vi "Begin.vi"(8 "error in (no error)":errorcluster, 9 "Left":T1, 10 "Right":T1, 11 "Pod Drive in":refnum<class "Pod Drive.lvclass">) -> (0 "error out":errorcluster, 3 "Pod Drive out":refnum<class "Pod Drive.lvclass">)   [LabVIEW 2018, in "Drive.lvlib" / "Pod Drive.lvclass"]
doc: "This VI holds the begin code"
uses:
  Pod Drive.lvclass
  Pod.ctl
  <vilib>/Rock Robotics/WPI/SafetyOutput/WPI_SafetyOutputConfigMenu.ctl
  Pod Drive.lvclass/Pod Drive.ctl
  <vilib>/Rock Robotics/WPI/RobotDrive/WPI_RobotDriveOpen2MotorWithExistingMotors.vi
  Drive.lvclass
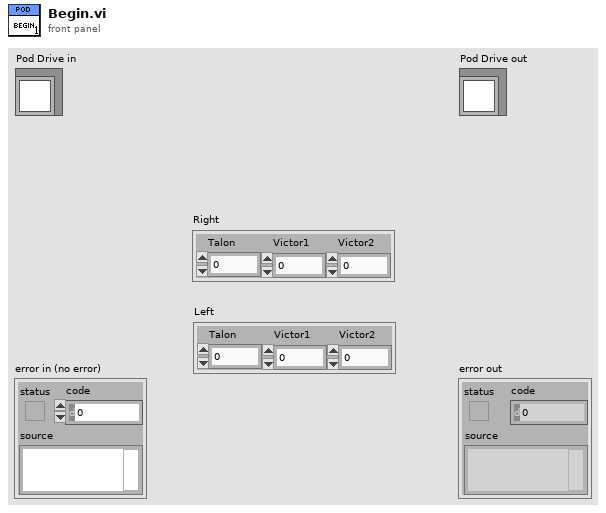
[diagram p1: front panel]
types:
  T1 = typedef "Drive.lvlib/Pod Drive.lvclass/Pod.ctl" = cluster{"Talon":u8, "Victor1":u8, "Victor2":u8}
  T2 = typedef "WPI_SafetyOutputConfigMenu.ctl" = enum16{"Enable", "Disable"}
  T3 = typedef "Drive.lvlib/Drive.lvclass/Drive Sensor Data.ctl" = cluster{"Drive Right Invert":bool, "Drive Right Sensor Phase":bool, "Drive Left Invert":bool, "Drive Left Sensor Phase":bool}
  T4 = typedef "WPI_MotorControlDeviceRef.ctl" = cluster{"DeviceStatus":errorcluster, "Type":T5, "PWM":cluster{"PWM Channel":T6, "DeadBand":T7}, "CAN":cluster{"Device Number":u8, "SetOutput VI Ref":variant, "GetOutput VI Ref":variant, "Enable VI Ref":variant, "Disable VI Ref":variant, "Data":variant}, "Invert":bool, "DIO PWM":cluster{"PWM \"Enable\" Channel":T6, "DIOChannel":T8, "PWM Rate":dbl}}
  T5 = typedef "WPI_MotorControlType.ctl" = enum16{"PWM", "CAN", "DIO PWM"}
  T6 = typedef "FPGA_DIOPWMChannel.ctl" = enum8{"PWM 0", "PWM 1", "PWM 2", "PWM 3", "PWM 4", "PWM 5", "PWM 6", "PWM 7", "PWM 8", "PWM 9", "PWM MXP 0", "PWM MXP 1", "PWM MXP 2", "PWM MXP 3", "PWM MXP 4", "PWM MXP 5", "PWM MXP 6", "PWM MXP 7", "PWM MXP 8", "PWM MXP 9", "Invalid"}
  T7 = typedef "WPI_PWMDeadband.ctl" = cluster{"Name":string, "maxPositivePwm":i32, "minPositivePwm":i32, "centerPwm":i32, "maxNegativePwm":i32, "minNegativePwm":i32, "angularRange":u16}
  T8 = typedef "FPGA_DIOChannel.ctl" = enum8{"DIO 0", "DIO 1", "DIO 2", "DIO 3", "DIO 4", "DIO 5", "DIO 6", "DIO 7", "DIO 8", "DIO 9", "DIO MXP 0", "DIO MXP 1", "DIO MXP 2", "DIO MXP 3", "DIO MXP 4", "DIO MXP 5", "DIO MXP 6", "DIO MXP 7", "DIO MXP 8", "DIO MXP 9", "DIO MXP 10", "DIO MXP 11", "DIO MXP 12", "DIO MXP 13", "DIO MXP 14", "DIO MXP 15", "SPI Port CS1", "SPI Port CS2", "SPI Port CS3", "SPI Port MISO", "SPI Port MOSI", "Invalid"}
  T9 = typedef "WPI_RobotDriveDevRef.ctl" = cluster{"DevStatus":errorcluster, "Motors[]":T4[], "Square Inputs":bool, "Max Output":dbl}
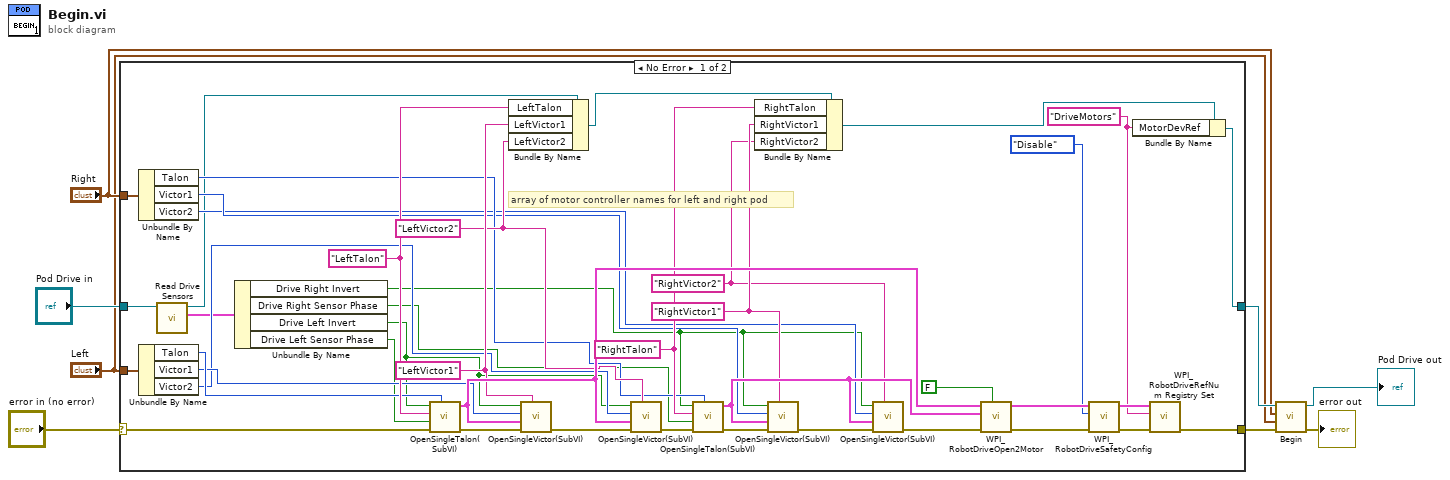
[diagram p0: block diagram]
diagram:
  n1 = case shown="No Error" "error in (no error)" {
    selector: "error in (no error)" -> [w28 w51]
    tunnel: [w24 w51] -> w6
    tunnel: [w27 w50] -> w4
    tunnel: "Pod Drive in" -> [w15 w50]
    tunnel: "Right" -> [w23 _]
    tunnel: "Left" -> [w22 _]
    frame No Error {
      w30 = "RightVictor2" ("RightVictor2")
      w31 = "RightVictor1" ("RightVictor1")
      w37 = "DriveMotors" ("refnum name")
      w26 = "RightTalon" ("RightTalon")
      w39 = "LeftVictor2" ("LeftVictor2")
      w40 = "LeftVictor1" ("LeftVictor1")
      w25 = "LeftTalon" ("LeftTalon")
      # "array of motor controller names for left and right pod"
      n2 = Unbundle By Name(w23) -> ("Talon"=w18:u8, "Victor1"=w17:u8, "Victor2"=w16:u8)
      n3 = Unbundle By Name(w22) -> ("Talon"=w21:u8, "Victor1"=w20:u8, "Victor2"=w19:u8)
      n4 = call-dynamic "Read Drive Sensors.vi"("Drive in"=w15) -> ("Drive Sensors"=w13:T3, "Drive out"=w14:refnum<class "Pod Drive.lvclass">)  [unwired: 8 in, 1 out]
      n5 = Unbundle By Name(w13) -> ("Drive Right Invert"=w9:bool, "Drive Right Sensor Phase"=w11:bool, "Drive Left Invert"=w10:bool, "Drive Left Sensor Phase"=w12:bool)
      n6 = call "OpenSingleTalon(SubVI).vi"("can_id"=w21, "error in (no error)"=w28, "sensor_phase"=w12, "refnum name"=w25, "invert"=w10) -> ("error out"=w43:errorcluster, "PhoenixMotorControlDevRef"=w41:T4)  [unwired: 5 in]
      n7 = Bundle By Name(cluster=w14, "LeftTalon"=w25, "LeftVictor1"=w40, "LeftVictor2"=w39) -> (w38:refnum<class "Pod Drive.lvclass">)
      n8 = call "OpenSingleVictor(SubVI).vi"("refnum name"=w40, "error in (no error)"=w43, "Master Controller to Follow"=w41, "Device Number"=w20, "Invert?"=w10) -> ("error out"=w42:errorcluster)  [unwired: 5 in, 1 out]
      n9 = call "OpenSingleVictor(SubVI).vi"("refnum name"=w39, "error in (no error)"=w42, "Master Controller to Follow"=w41, "Device Number"=w19, "Invert?"=w10) -> ("error out"=w35:errorcluster)  [unwired: 5 in, 1 out]
      n10 = call "OpenSingleTalon(SubVI).vi"("can_id"=w18, "error in (no error)"=w35, "sensor_phase"=w11, "refnum name"=w26, "invert"=w9) -> ("error out"=w34:errorcluster, "PhoenixMotorControlDevRef"=w32:T4)  [unwired: 5 in]
      n11 = Bundle By Name(cluster=w38, "RightTalon"=w26, "RightVictor1"=w31, "RightVictor2"=w30) -> (w36:refnum<class "Pod Drive.lvclass">)
      n12 = call "OpenSingleVictor(SubVI).vi"("refnum name"=w31, "error in (no error)"=w34, "Master Controller to Follow"=w32, "Device Number"=w17, "Invert?"=w9) -> ("error out"=w33:errorcluster)  [unwired: 5 in, 1 out]
      n13 = call "OpenSingleVictor(SubVI).vi"("refnum name"=w30, "error in (no error)"=w33, "Master Controller to Follow"=w32, "Device Number"=w16, "Invert?"=w9) -> ("error out"=w29:errorcluster)  [unwired: 5 in, 1 out]
      n14 = call-poly <vilib>:"WPI_RobotDriveOpen2Motor.vi"("Square Inputs"=FALSE, "error in (no error)"=w29, "Right Motor Dev Ref"=w32, "Left Motor Dev Ref"=w41) -> ("error out"=w49:errorcluster, "RobotDriveDevRef"=w47:T9)  [unwired: 6 in]
      n15 = call <vilib>:"WPI_RobotDriveSafetyConfig.vi"("error in (no error)"=w49, "mode"=WPI_SafetyOutputConfigMenu."Disable", "RobotDriveDevRef"=w47) -> ("error out"=w48:errorcluster, "RobotDriveDevRef"=w46:T9)  [unwired: 7 in]
      n16 = Bundle By Name(cluster=w36, "MotorDevRef"=w37) -> (w27:refnum<class "Pod Drive.lvclass">)
      n17 = call <vilib>:"WPI_RobotDriveRefNum Registry Set.vi"("error in (no error)"=w48, "refnum name"=w37, "RobotDriveDevRef"=w46) -> ("error out"=w24:errorcluster)  [unwired: 7 in, 1 out]
    }
    frame Error {
    }
  }
  n18 = call-parent "Begin.vi"("error in (no error)"=w6, "Left"="Left", "Right"="Right", "Drive in"=w4) -> ("error out"=→"error out":errorcluster, "Drive out"=→"Pod Drive out":refnum<class "Pod Drive.lvclass">)  [unwired: 6 in]
